vi "random_games.vi"() -> ()   [LabVIEW 2021]
uses:
  <vilib>/numeric/Random Number (Range) DBL.vi
panel:
  out "Waveform Graph":i32[][](graph)
  out "Points B":dbl
  out "Points A":dbl
  out "Random Number B":dbl
  out "Random Number A":dbl
  out "Number of Iterations":dbl
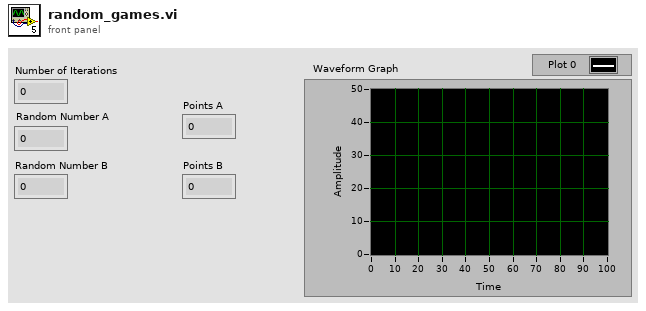
[diagram p1: front panel]
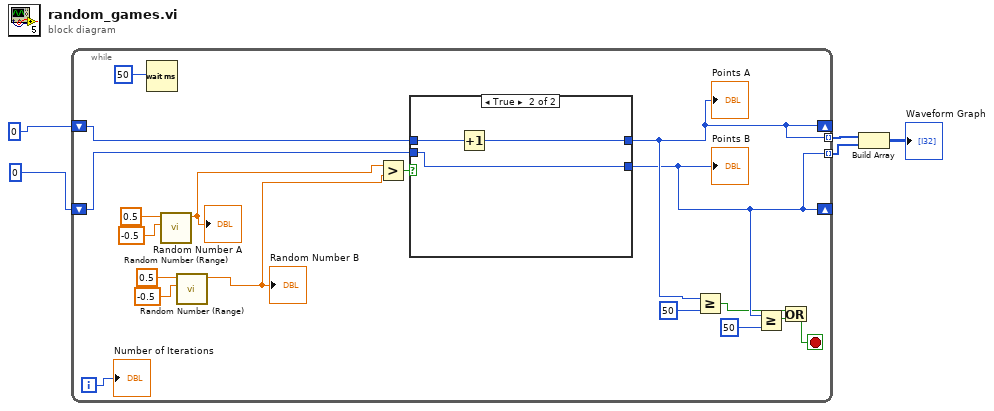
[diagram p0: block diagram]
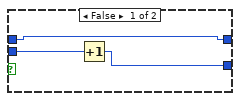
[diagram p2: hidden frame]
diagram:
  n1 = while {
    shift-right: [w10] -> _
    shift-left: 0 -> [w15]
    shift-right: [w11] -> _
    shift-left: 0 -> [w14]
    tunnel: [w11] -> w2 mode=indexing
    tunnel: [w10] -> w1 mode=indexing
    i -> [w6]
    stop <- w9 stop-if-true
    n2 = Wait (ms)(milliseconds to wait=50) -> ()  [unwired: 1 out]
    n3 = call-poly <vilib>:"Random Number (Range).vi"("lower bound (0)"=-0.5, "upper bound (100)"=0.5) -> ("number"=w17:dbl)  [unwired: 9 in]
    "Random Number A" <- w17
    n4 = call-poly <vilib>:"Random Number (Range).vi"("lower bound (0)"=-0.5, "upper bound (100)"=0.5) -> ("number"=w16:dbl)  [unwired: 9 in]
    "Random Number B" <- w16
    n5 = Greater?(x=w17, y=w16) -> (0:w18:bool)
    n6 = case shown="True" w18 {
      tunnel: w14 -> [w24 w29]
      tunnel: [w24 w28] -> w11
      tunnel: w15 -> [w26 w27]
      tunnel: [w25 w27] -> w10
      frame False {
        n7 = Increment(x=w26) -> (x+1=w25:i32)
      }
      frame True {
        n8 = Increment(x=w29) -> (x+1=w28:i32)
      }
    }
    "Points A" <- w11
    "Points B" <- w10
    n9 = Greater Or Equal?(x=w11, y=50) -> (x >= y?=w8:bool)
    n10 = Greater Or Equal?(x=w10, y=50) -> (x >= y?=w7:bool)
    n11 = Or(x=w8, y=w7) -> (x .or. y?=w9:bool)
    "Number of Iterations" <- w6
  }
  n12 = Build Array(w2, w1) -> (→"Waveform Graph":i32[][])
